vi "User Message Received.vi"(0 "Diplom in":refnum<class "Diplom.lvclass">, 5 "Message":refnum<class "Message.lvclass">, 11 "Error in":errorcluster caption="Error in (no error)") -> (4 "Diplom out":refnum<class "Diplom.lvclass">, 15 "Error out":errorcluster)   [LabVIEW 2018, in "HOG Diplom.lvlib" / "Diplom.lvclass"]
doc: "This VI runs whenever the Actor Core receives a message. Any messages not handled here are simply discarded.\n\n<B>You should not invoke the Call Parent Method node when adding this override.</B>\n\nSteen Schmidt\nGPower\n8/5 2017"
uses:
  Diplom.lvclass
  <vilib>/GPower/Message/Library/Message Class/Message.lvclass
  <vilib>/GPower/Message/Library/Message Class/Message.lvclass/Message.ctl
  <vilib>/GPower/Dictionary/Library/Dictionary Class/Dictionary.lvclass
  <vilib>/Utility/NIReport.llb/Report Type.ctl
  <vilib>/GPower/Message With Data/Library/Data Message Class/Data Message.lvclass/Data Message.ctl
  Diplom.lvclass/Diplom.ctl
  24e689c4-c721-4ec3-80a5-68a2c90e728a.vi
  4c1fff5f-4e0d-42da-941c-ad3010e70a5f.vi
  16e9147c-62b6-4527-a28f-6dc7c6610bc8.vi
  00c7285f-6734-4c39-b096-9109ac4122e9.vi
  <vilib>/GPower/Message With Data/Library/Data Message Class/Accessors/Get Data.vi
  <vilib>/GPower/Dictionary/Library/Dictionary Class/Get/Get Path.vi
  <vilib>/addons/_office/word.llb/Word Find & Replace (str).vi
  <vilib>/GPower/Message With Data/Library/Data Message Class/Data Message.lvclass
  <vilib>/Utility/NIReport.llb/NI_report.lvclass
  <vilib>/Utility/NIReport.llb/NI_ReportGenerationCore.lvlib
  <vilib>/addons/_office/NI_ReportGenerationToolkit.lvlib
  <vilib>/Utility/NIReport.llb/Word/NI_Word.lvclass
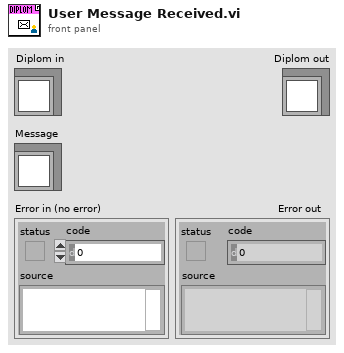
[diagram p1: front panel]
types:
  T1 = typedef "NI_ReportGenerationCore.lvlib/Report Type.ctl" = enum16{"HTML", "Word", "Excel"}
  T2 = enum16{"maximized", "minimized", "normal", "no change"}
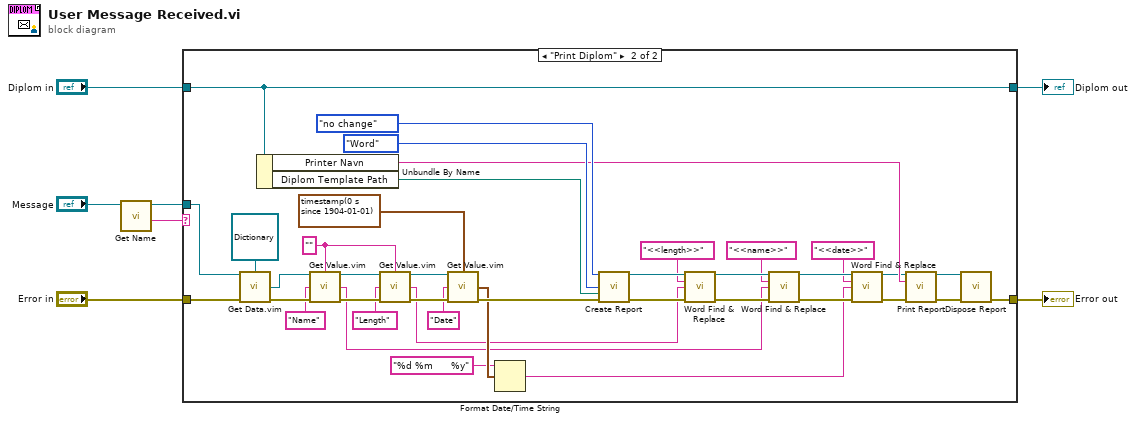
[diagram p0: block diagram]
diagram:
  n1 = call <vilib>:"Get Name.vi"("Message in"="Message") -> ("Name"=w6:string, "Message out"=w5:refnum<class "Message.lvclass">)  [unwired: 9 in]
  n2 = case shown="\"Print Diplom\"" w6 {
    tunnel: w5 -> [_ w48]
    tunnel: "Error in" -> [w9 w47]
    tunnel: [w9 w13] -> w3
    tunnel: "Diplom in" -> [w8 w10]
    tunnel: [w8 w10] -> w1
    frame Default {
    }
    frame "Print Diplom" {
      w38 = ""
      n3 = call "Get Data.vim"("Data Message in"=w48, "Data Type"=refnum<class "Dictionary.lvclass"> refnum ("New Dictionary"), "Error in"=w47) -> ("Data"=w44:refnum<class "Dictionary.lvclass">, "Error out"=w45:errorcluster)  [unwired: 10 in, 1 out]
      n4 = Unbundle By Name(w10) -> ("Printer Navn"=w15:string, "Diplom Template Path"=w34:path)
      n5 = call "Get Value.vim"("Dictionary in"=w44, "Value Type"=w38, "Key Path"="Name", "Error in"=w45) -> ("Dictionary out"=w40:refnum<class "Dictionary.lvclass">, "Value"=w17:string, "Error out"=w42:errorcluster)  [unwired: 9 in]
      n6 = call "Get Value.vim"("Dictionary in"=w40, "Value Type"=w38, "Key Path"="Length", "Error in"=w42) -> ("Dictionary out"=w39:refnum<class "Dictionary.lvclass">, "Value"=w18:string, "Error out"=w41:errorcluster)  [unwired: 9 in]
      n7 = call "Get Value.vim"("Dictionary in"=w39, "Value Type"=timestamp(0 s since 1904-01-01) ("current time"), "Key Path"="Date", "Error in"=w41) -> ("Value"=w21:timestamp, "Error out"=w33:errorcluster)  [unwired: 9 in, 1 out]
      n8 = Format Date/Time String(time format string (%c)="%d %m      %y", seconds (now)=w21) -> (date/time string=w19:string)  [unwired: 1 in]
      n9 = call <vilib>:"Create Report.vi"("window state (normal)"=T2."no change", "report type"=Report_Type."Word", "template (empty)"=w34, "error in (no error)"=w33) -> ("report out"=w28:refnum<class "NI_report.lvclass">, "error out"=w31:errorcluster)  [unwired: 10 in]
      n10 = call-poly <vilib>:"Word Find & Replace.vi"("report in"=w28, "find what?"="<<length>>", "replace with"=w18, "error in (no error)"=w31) -> ("report out"=w27:refnum<class "NI_report.lvclass">, "error out"=w30:errorcluster)  [unwired: 9 in, 1 out]
      n11 = call-poly <vilib>:"Word Find & Replace.vi"("report in"=w27, "find what?"="<<name>>", "replace with"=w17, "error in (no error)"=w30) -> ("report out"=w26:refnum<class "NI_report.lvclass">, "error out"=w29:errorcluster)  [unwired: 9 in, 1 out]
      n12 = call-poly <vilib>:"Word Find & Replace.vi"("report in"=w26, "find what?"="<<date>>", "replace with"=w19, "error in (no error)"=w29) -> ("report out"=w11:refnum<class "NI_report.lvclass">, "error out"=w16:errorcluster)  [unwired: 9 in, 1 out]
      n13 = call-dynamic "Print Report.vi"("report in"=w11, "printer name (default)"=w15, "error in (no error)"=w16) -> ("report out"=w12:refnum<class "NI_report.lvclass">, "error out"=w14:errorcluster)  [unwired: 11 in]
      n14 = call-dynamic "Dispose Report.vi"("report in"=w12, "error in (no error)"=w14) -> ("error out"=w13:errorcluster)  [unwired: 13 in]
    }
  }
  "Diplom out" <- w1
  "Error out" <- w3
